vi "T16.vi"(2 "Parametry Ziemi":T1={"a - półoś duża"=6378137.0, "b - półoś mała"=6356752.3141999999998} {"b - półoś mała" format="%_20f"; "a - półoś duża" format="%_20g"}, 3 "fi'":ext) -> (7 "T16":ext)   [LabVIEW 2015, in "Biblioteka moduł map v3.lvlib" / "Konwersja wsp.lvlib" / "UTM.lvlib" / "Konwersja z UTM na wsp geograficzne.lvlib"]
uses:
  Konwersja z UTM na wsp geograficzne.lvlib
  UTM.lvlib
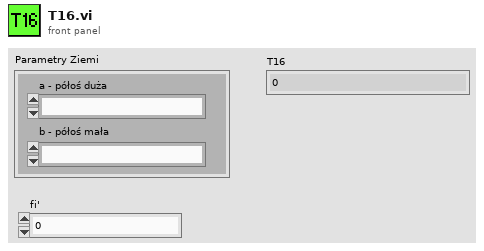
[diagram p1: front panel]
types:
  T1 = cluster{"a - półoś duża":ext, "b - półoś mała":ext}
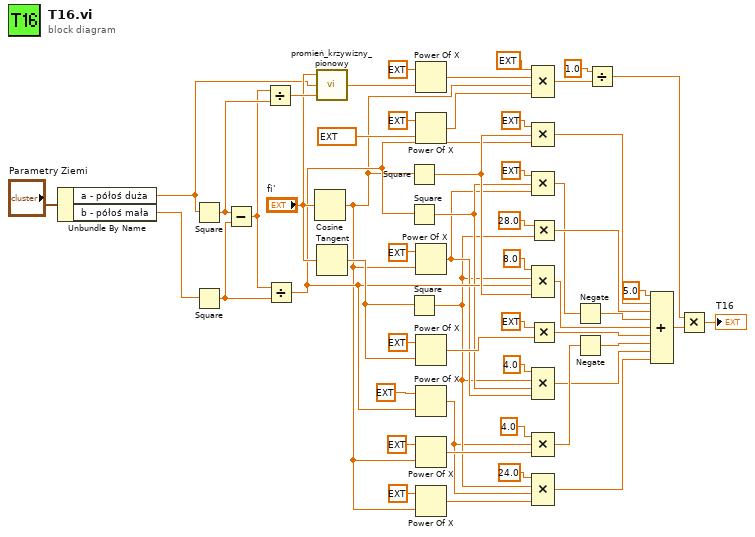
[diagram p0: block diagram]
diagram:
  n1 = Unbundle By Name("Parametry Ziemi") -> ("a - półoś duża"=w2:ext, "b - półoś mała"=w1:ext)
  n2 = Square(x=w2) -> (x^2=w55:ext)
  n3 = Square(x=w1) -> (x^2=w38:ext)
  n4 = Subtract(x=w55, y=w38) -> (x-y=w39:ext)
  n5 = Divide(x=w39, y=w55) -> (x/y=w54:ext)
  n6 = Divide(x=w39, y=w38) -> (x/y=w18:ext)
  n7 = Cosine(x="fi'") -> (cos(x)=w6:ext)
  n8 = call "promień_krzywizny_pionowy.vi"("e^2"=w54, "a"=w2, "fi[rad]"="fi'") -> ("Promien krzywizny równoleżnika"=w51:dbl)  [unwired: 2 in]
  n9 = Tangent(1:"fi'") -> (0:w26:ext)
  n10 = Square(x=w6) -> (x^2=w27:ext)
  n11 = Square(x=w18) -> (x^2=w14:ext)
  n12 = Square(x=w26) -> (x^2=w9:ext)
  n13 = Power Of X(1:w51, 2:ext 5.0 ("y")) -> (0:w49:ext)
  n14 = Power Of X(1:ext 0.9996 ("k0"), 2:ext 5.0 ("y")) -> (0:w45:ext)
  n15 = Power Of X(1:w6, 2:ext 4.0 ("y")) -> (0:w13:ext)
  n16 = Power Of X(1:w26, 2:ext 4.0 ("y")) -> (0:w24:ext)
  n17 = Power Of X(1:w18, 2:ext 3.0 ("y")) -> (0:w8:ext)
  n18 = Power Of X(1:w6, 2:ext 6.0 ("y")) -> (0:w16:ext)
  n19 = Power Of X(1:w6, 2:ext 6.0 ("y")) -> (0:w7:ext)
  n20 = Multiply(x=28.0, y=w9) -> (x*y=w34:ext)
  n21 = Multiply(x=ext 24.0, y=w24) -> (x*y=w22:ext)
  n22 = Compound Arithmetic op=MULTIPLY(ext 120.0 ("value"), w49, w6, w45) -> (w52:ext)
  n23 = Compound Arithmetic op=MULTIPLY(ext 6.0 ("value"), w27, w18) -> (w37:ext)
  n24 = Compound Arithmetic op=MULTIPLY(ext 3.0 ("value"), w14, w13) -> (w32:ext)
  n25 = Compound Arithmetic op=MULTIPLY(8.0 ("value"), w9, w18, w27) -> (w29:ext)
  n26 = Compound Arithmetic op=MULTIPLY(4.0 ("value"), w9, w14, w13) -> (w12:ext)
  n27 = Compound Arithmetic op=MULTIPLY(4.0 ("value"), w8, w16) -> (w21:ext)
  n28 = Compound Arithmetic op=MULTIPLY(24.0 ("value"), w9, w8, w7) -> (w11:ext)
  n29 = Negate(x=w32) -> (-x=w31:ext)
  n30 = Negate(x=w21) -> (-x=w20:ext)
  n31 = Divide(x=1.0, y=w52) -> (x/y=w44:ext)
  n32 = Compound Arithmetic op=ADD(5.0 ("value"), w37, w34, w31, w29, w22, w20, w12, w11) -> (w43:ext)
  n33 = Multiply(x=w44, y=w43) -> (x*y=→"T16":ext)
